vi "Acquisition Message Loop.vi"(0 "Files d'attente de messages":T2, 5 "Notificateur de données":refnum<notifier>, 9 "File d'attente de données":refnum<queue>, 11 "error in (no error)":T1 caption="entrée d'erreur (pas d'erreur)") -> (15 "error out":T1 caption="sortie d'erreur")   [LabVIEW 2018, in "Acquisition.lvlib"]
doc: "Boucle de message pour traiter les messages concernant l'acquisition de données du matériel."
uses:
  Acquisition.lvlib
  support/Message Queue/All Message Queues.ctl
  support/Message Queue/Message Cluster.ctl
  Hardware Configuration.ctl
  Signal Type.ctl
  Acquisition State.ctl
  support/Message Queue/Enqueue Message (Single).vi
  <vilib>/Utility/error.llb/Error Cluster From Error Code.vi
  <vilib>/ErrorRing/Error Ring.xnode
  support/Message Queue/Message Queue.lvlib
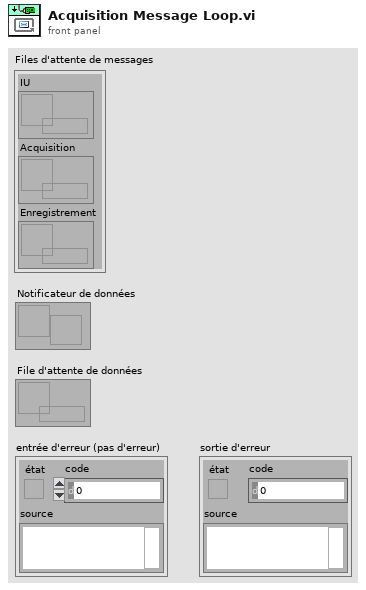
[diagram p1: front panel]
types:
  T1 = cluster{"état":bool, "code":i32, "source":string}
  T2 = typedef "Message Queue.lvlib/All Message Queues.ctl" = cluster{"IU":refnum<queue>, "Acquisition":refnum<queue>, "Enregistrement":refnum<queue>}
  T3 = typedef "Acquisition.lvlib/Hardware Configuration.ctl" = cluster{"Refnum de matériel <À remplacer>":string, "Type de signal <À remplacer>":T4}
  T4 = typedef "Acquisition.lvlib/Signal Type.ctl" = enum16{"Sine Wave", "Square with Noise", "Signal triangulaire", "Simulation DAQ"}
  T5 = typedef "Acquisition.lvlib/Acquisition State.ctl" = enum16{"Idle", "Acquiring"}
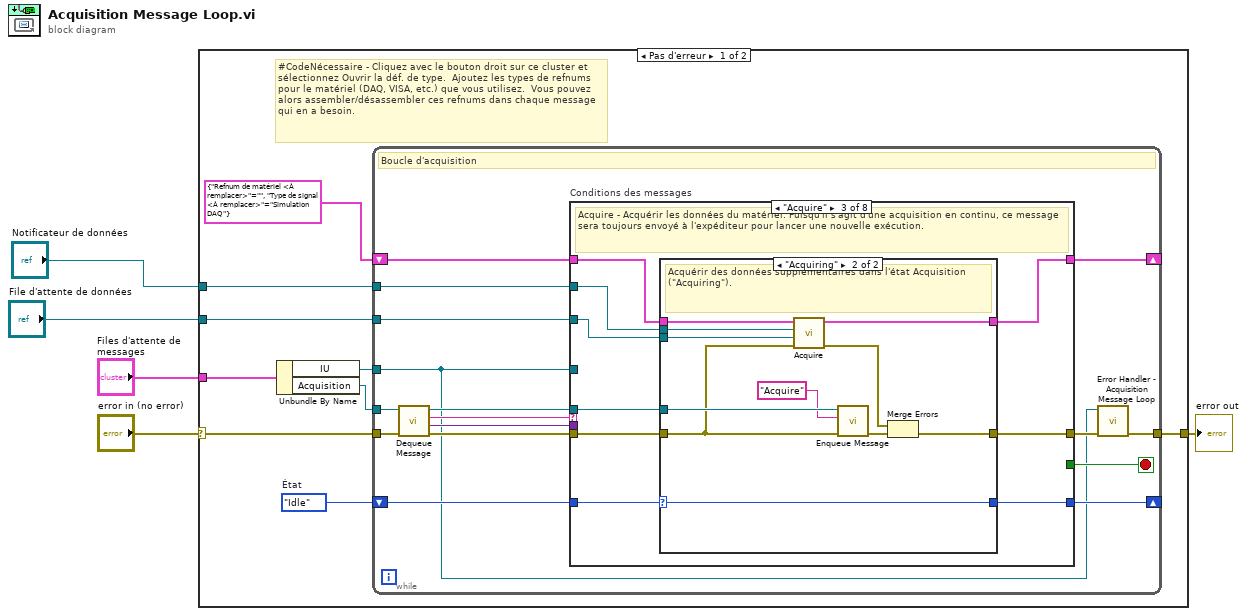
[diagram p0: block diagram]
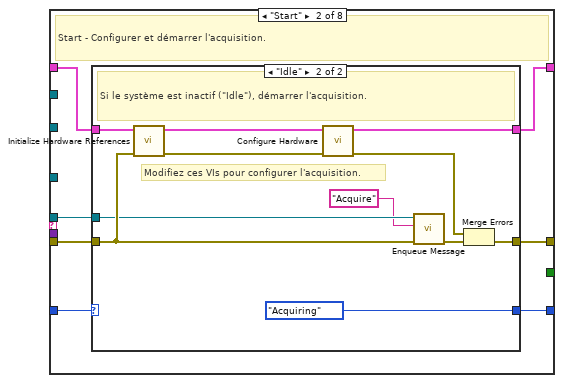
[diagram p3: hidden frame]
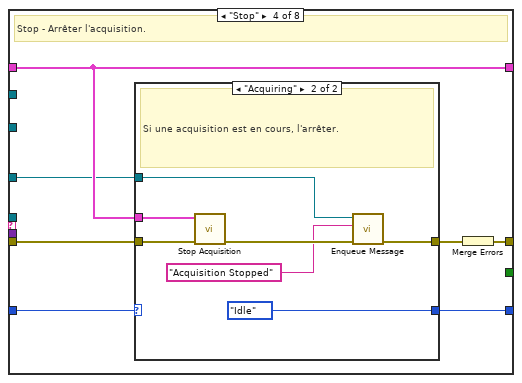
[diagram p6: hidden frame]
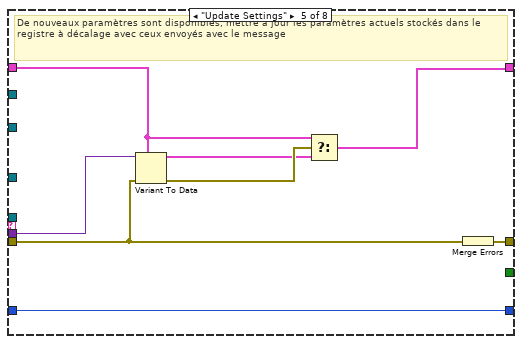
[diagram p8: hidden frame]
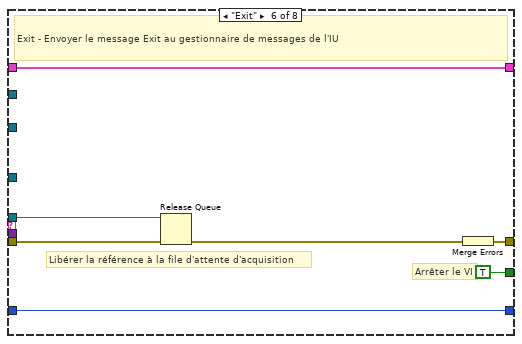
[diagram p9: hidden frame]
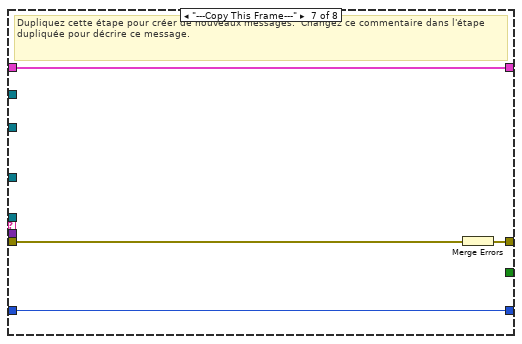
[diagram p10: hidden frame]
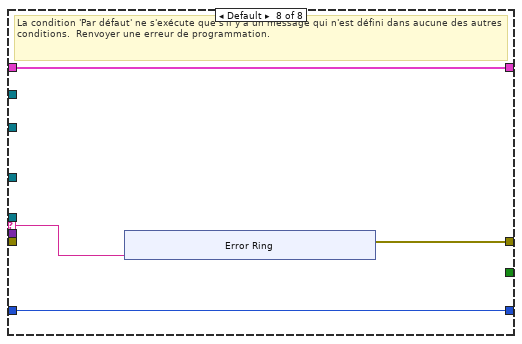
[diagram p11: hidden frame]
diagram:
  n1 = case shown="Pas d'erreur" "error in (no error)" {
    selector: "error in (no error)" -> [w10 w124]
    tunnel: "Files d'attente de messages" -> [w14 _]
    tunnel: [w12 w124] -> w4
    tunnel: "Notificateur de données" -> [w8 _]
    tunnel: "File d'attente de données" -> [w7 _]
    frame No Error {
      w6 = Acquisition_State."Idle"  # État
      # "#CodeNécessaire - Cliquez avec le bouton droit sur ce cluster et sélectionnez Ouvrir la déf. de type.  Ajoutez les types de refnums pour le matériel (DAQ, VISA, etc.) que vous utilisez.  Vous pouvez alors assembler/désassembler ces refnums dans chaque message qui en a besoin."
      n2 = Unbundle By Name(w14) -> ("IU"=w9:refnum<queue>, "Acquisition"=w13:refnum<queue>)
      n3 = while {
        tunnel: w13 -> [w23]
        shift-right: [w29] -> _
        shift-left: T3 {"Refnum de matériel <À remplacer>"="", "Type de signal <À remplacer>"=enum."Simulation DAQ"} ("Data Cluster") -> [w30]
        tunnel: w9 -> [w15]
        tunnel: w8 -> [w22]
        tunnel: w7 -> [w21]
        shift-right: [w19] -> _
        shift-left: w6 -> [w20]
        tunnel: w10 -> [w27]
        tunnel: [w18] -> w12
        stop <- w28 stop-if-true
        # "Boucle d'acquisition"
        n4 = call "Dequeue Message.vi"("error in (no error)"=w27, "File d'attente de messages"=w23) -> ("error out"=w26:T1, "Données de message"=w24:variant, "Message"=w25:string, "File d'attente de message dup."=w16:refnum<queue>)  [unwired: 6 in]
        n5 = case "Conditions des messages" shown="\"Acquire\"" w25 {
          selector: w25 -> [_ _ _ _ _ _ _ w113]
          tunnel: w16 -> [_ w37 w62 _ _ w103 _ _]
          tunnel: w26 -> [w33 w38 w61 w83 w95 w105 w112 _]
          tunnel: [w33 w40 w63 w84 w101 w107 w110 w114] -> w17
          tunnel: w30 -> [w32 w39 w59 w81 w97 w106 w111 w116]
          tunnel: [w32 w36 w60 w81 w96 w106 w111 w116] -> w29
          tunnel: [_ _ _ _ _ TRUE _ _] -> w28
          tunnel: w24 -> [_ _ _ _ w100 _ _ _]
          tunnel: w15 -> [_ _ _ w78 _ _ _ _]
          tunnel: w22 -> [_ _ w58 _ _ _ _ _]
          tunnel: w21 -> [_ _ w57 _ _ _ _ _]
          tunnel: w20 -> [w31 w34 w55 w80 w94 w102 w109 w115]
          tunnel: [w31 w35 w56 w79 w94 w102 w109 w115] -> w19
          frame "Initialize" {
            # "Initialize - À ce point-ci, Initialize n'a aucune fonction.  L'initialisation du matériel a lieu dans le message 'Start'."
          }
          frame "Start" {
            # "Start - Configurer et démarrer l'acquisition."
            n6 = case shown="\"Idle\"" w34 {
              selector: w34 -> [w41 _]
              tunnel: [w42 w54] -> w40
              tunnel: w39 -> [w43 w53]
              tunnel: w38 -> [w42 w52]
              tunnel: w37 -> [_ w50]
              tunnel: [w43 w46] -> w36
              tunnel: [w41 Acquisition_State."Acquiring" ("Acquisition State")] -> w35
              frame "Acquiring" {
                # "L'acquisition est déjà en cours. Ignorer le message \"Start\"."
              }
              frame "Idle" {
                # "Modifiez ces VIs pour configurer l'acquisition."
                # "Si le système est inactif (\"Idle\"), démarrer l'acquisition."
                n7 = call "Initialize Hardware References.vi"("error in (no error)"=w52, "Ressources matérielles en entrée"=w53) -> ("error out"=w49:T1, "Ressources matérielles en sortie"=w47:T3)  [unwired: 8 in]
                n8 = call "Configure Hardware.vi"("error in (no error)"=w49, "Ressources matérielles en entrée"=w47) -> ("error out"=w48:T1, "Ressources matérielles en sortie"=w46:T3)  [unwired: 8 in]
                n9 = call-poly "Enqueue Message.vi"("error in (no error)"=w52, "Message"="Acquire", "File d'attente de messages"=w50) -> ("error out"=w51:T1)  [unwired: 7 in, 1 out]
                n10 = Merge Errors(w48, w51) -> (w54:errorcluster)
              }
            }
          }
          frame "Acquire" {
            # "Acquire - Acquérir les données du matériel. Puisqu'il s'agit d'une acquisition en continu, ce message sera toujours envoyé à l'expéditeur pour lancer une nouvelle exécution."
            n11 = case shown="\"Acquiring\"" w55 {
              selector: w55 -> [w64 w68]
              tunnel: [w65 w77] -> w63
              tunnel: w62 -> [_ w75]
              tunnel: w61 -> [w65 w67]
              tunnel: [w66 w73] -> w60
              tunnel: w59 -> [w66 w72]
              tunnel: w58 -> [_ w70]
              tunnel: w57 -> [_ w69]
              tunnel: [w64 w68] -> w56
              frame "Idle" {
                # "Ignorer les messages \"Acquire\" quand l'acquisition est inactive."
              }
              frame "Acquiring" {
                # "Acquérir des données supplémentaires dans l'état Acquisition (\"Acquiring\")."
                n12 = call "Acquire.vi"("error in (no error)"=w67, "File d'attente de données"=w69, "Notificateur de données"=w70, "Ressources matérielles en entrée"=w72) -> ("error out"=w74:T1, "Ressources matérielles en sortie"=w73:T3)  [unwired: 6 in]
                n13 = call-poly "Enqueue Message.vi"("error in (no error)"=w67, "Message"="Acquire", "File d'attente de messages"=w75) -> ("error out"=w76:T1)  [unwired: 7 in, 1 out]
                n14 = Merge Errors(w74, w76) -> (w77:errorcluster)
              }
            }
          }
          frame "Stop" {
            # "Stop - Arrêter l'acquisition."
            n15 = case shown="\"Acquiring\"" w80 {
              selector: w80 -> [w85 _]
              tunnel: w83 -> [w86 w93]
              tunnel: [w86 w89] -> w82
              tunnel: w81 -> [_ w91]
              tunnel: [w85 Acquisition_State."Idle" ("State")] -> w79
              tunnel: w78 -> [_ w88]
              frame "Idle" {
                # "Le système est déjà inactif. Ignorer le message \"Stop\"."
              }
              frame "Acquiring" {
                # "Si une acquisition est en cours, l'arrêter."
                n16 = call "Stop Acquisition.vi"("error in (no error)"=w93, "Ressources matérielles en entrée"=w91) -> ("error out"=w92:T1)  [unwired: 9 in]
                n17 = call-poly "Enqueue Message.vi"("error in (no error)"=w92, "Message"="Acquisition Stopped", "File d'attente de messages"=w88) -> ("error out"=w89:T1)  [unwired: 7 in, 1 out]
              }
            }
            n18 = Merge Errors(w82) -> (w84:errorcluster)
          }
          frame "Update Settings" {
            # "De nouveaux paramètres sont disponibles, mettre à jour les paramètres actuels stockés dans le registre à décalage avec ceux envoyés avec le message"
            n19 = Variant To Data(error in=w95, type=w97, Variant=w100) -> (data=w98:T3, error out=w99:errorcluster)
            n20 = Select(t=w97, s=w99, f=w98) -> (s? t:f=w96:T3)
            n21 = Merge Errors(w95) -> (w101:errorcluster)
          }
          frame "Exit" {
            # "Libérer la référence à la file d'attente d'acquisition"
            # "Arrêter le VI"
            # "Exit - Envoyer le message Exit au gestionnaire de messages de l'IU"
            n22 = Release Queue(queue=w103, error in (no error)=w105) -> (error out=w104:errorcluster)  [unwired: 1 in, 2 out]
            n23 = Merge Errors(w104) -> (w107:errorcluster)
          }
          frame "---Copy This Frame---" {
            # "Dupliquez cette étape pour créer de nouveaux messages.  Changez ce commentaire dans l'étape dupliquée pour décrire ce message."
            n24 = Merge Errors(w112) -> (w110:errorcluster)
          }
          frame Default {
            # "La condition 'Par défaut' ne s'exécute que s'il y a un message qui n'est défini dans aucune des autres conditions.  Renvoyer une erreur de programmation."
            n25 = xnode ("Error Ring")("paramètre 0"=w113) -> ("sortie d'erreur"=w114:errorcluster)
          }
        }
        n26 = call "Error Handler - Acquisition Message Loop.vi"("error in (no error)"=w17, "File d'attente de messages"=w15) -> ("erreur en entrée dup."=w18:T1)  [unwired: 8 in, 1 out]
      }
    }
    frame Error {
    }
  }
  "error out" <- w4
